vi "Strip out Unused Tests.vi"(8 "error in (no error)":errorcluster, 10 "Test to remain":string, 11 "runs":T1[](array[typedef])) -> (0 "error out":errorcluster, 3 "runs":T1[](array[typedef]))   [LabVIEW 2011]
uses:
  www/cgi-bin/_cgi-lib/TDM_INDEX Record.ctl
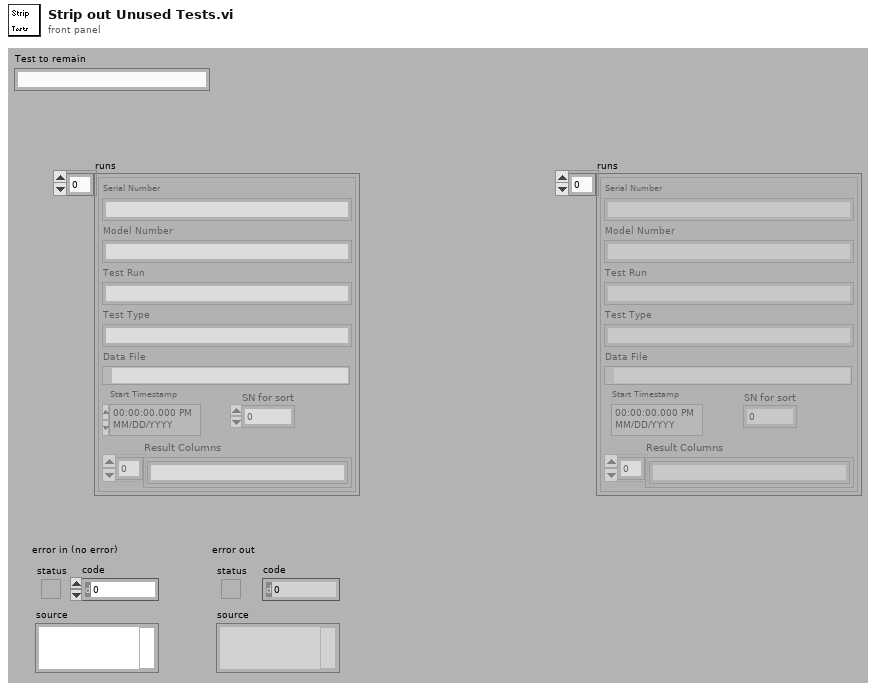
[diagram p1: front panel]
types:
  T1 = typedef "TDM_INDEX Record.ctl" = cluster{"Model Number":string, "SN for sort":i32, "Test Type":string, "Test Run":string, "Serial Number":string, "Start Timestamp":timestamp, "Data File":path, "Result Columns":string[]}
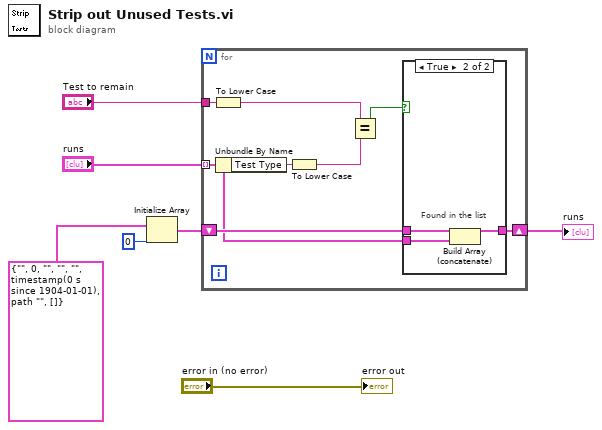
[diagram p0: block diagram]
diagram:
  n1 = Initialize Array(T1 {"Model Number"="", "SN for sort"=0, "Test Type"="", "Test Run"="", "Serial Number"="", "Start Timestamp"=timestamp(0 s since 1904-01-01), "Data File"=path "", "Result Columns"=[]} ("TDM_INDEX Record"), 0) -> (w5:T1[])
  n2 = for {
    shift-right: [w12] -> w2
    shift-left: w5 -> [w13]
    tunnel: "runs" -> [w11] mode=indexing
    tunnel: "Test to remain" -> [w15]
    n3 = To Lower Case(string=w15) -> (all lower case string=w10:string)
    n4 = Unbundle By Name(w11) -> ("Test Type"=w14:string)
    n5 = To Lower Case(string=w14) -> (all lower case string=w9:string)
    n6 = Equal?(x=w10, y=w9) -> (x = y?=w8:bool)
    n7 = case shown="True" w8 {
      tunnel: w13 -> [w16 w19]
      tunnel: [w16 w18] -> w12
      tunnel: w11 -> [_ w17]
      frame False {
        # "Didnt' find it ..."
      }
      frame True {
        # "Found in the list"
        n8 = Build Array (concatenate)(w19, w17) -> (w18:T1[])
      }
    }
  }
  "runs" <- w2
  "error out" <- "error in (no error)"
